vi "Compute Convex Fast Hull.vi"(2 "Bounding Rectangle (Entire Array)":T2={"Left"=-1, "Top"=-1, "Right"=-1, "Bottom"=-1}, 3 "Data":u16[][](array[numeric]), 4 "Center of Mass (0, 0)":T1) -> (0 "Interior":T1[](array[typedef]), 1 "Hull":T1[](array[typedef]))   [LabVIEW 2018, in "Video Cam Processor.lvclass"]
uses:
  Video Cam Processor.lvclass
  Private/Hull Point STYP.ctl
  Shared/Graham Scan/Graham Scan Bounding Rectangle STYP.ctl
  0152be87-d5b1-4a61-b902-843b2f58f9da.vi
  a4750f4a-c86b-4402-9379-9284bf635716.vi
  eb0064ed-dfcb-4dbb-84a7-5f2da3a78c84.vi
  2de1e9ff-1ea0-4ee2-97ee-32f0ea305ab5.vi
  ab02dc5e-4995-41ed-abd7-7908662af6ba.vi
  6afddc17-1598-4bdd-b49e-99777c4027e1.vi
  1da664a8-6403-49de-8289-c04fd4f99e1f.vi
  d6c0e748-e52f-41a4-ae1e-f13c5fdb461c.vi
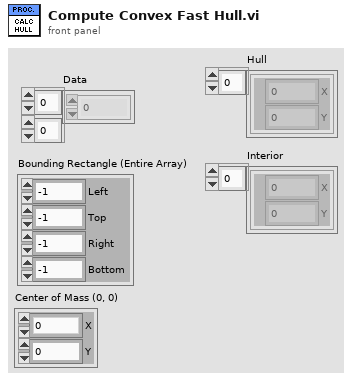
[diagram p1: front panel]
types:
  T1 = typedef "Video Cam Processor.lvclass/Hull Point STYP.ctl" = cluster{"X":i32, "Y":i32}
  T2 = typedef "Graham Scan Bounding Rectangle STYP.ctl" = cluster{"Left":i32, "Top":i32, "Right":i32, "Bottom":i32}
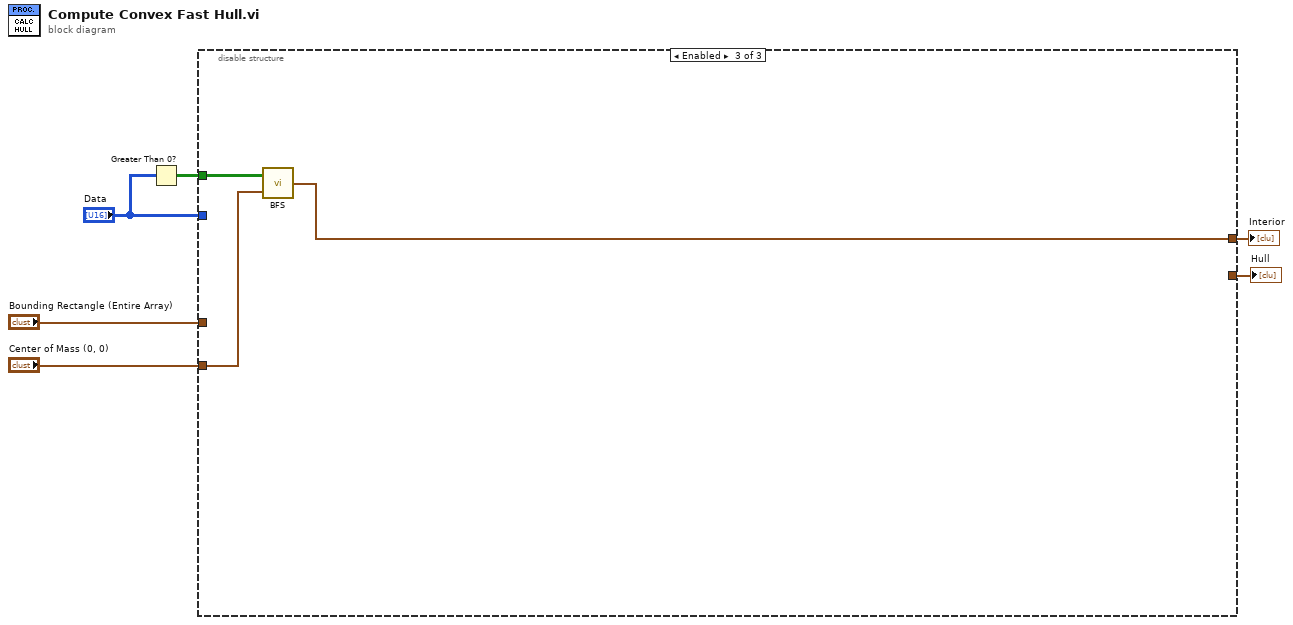
[diagram p0: block diagram]
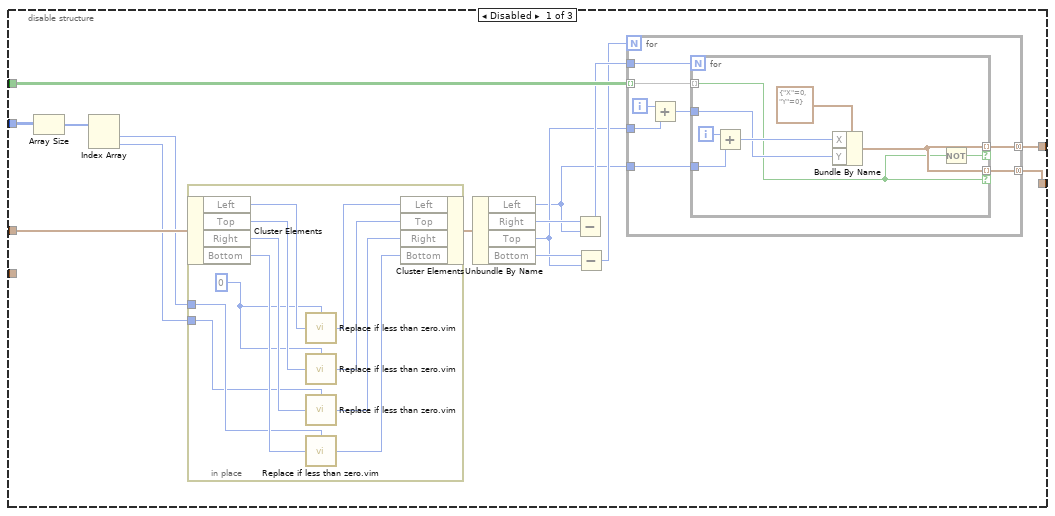
[diagram p2: hidden frame]
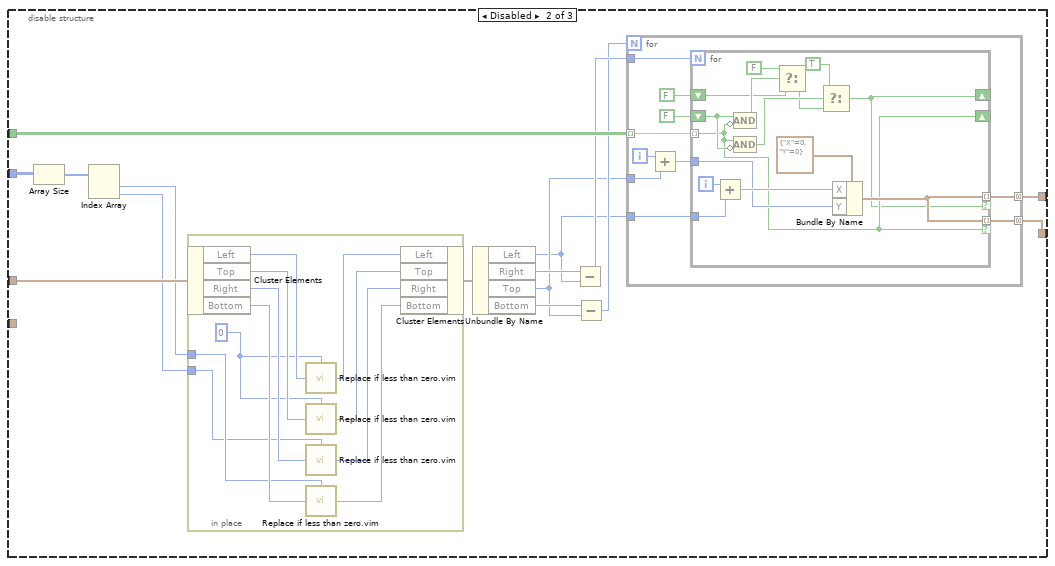
[diagram p3: hidden frame]
diagram:
  n1 = Greater Than 0?(x="Data") -> (x > 0?=w4:bool[][])
  n2 = disable-structure shown="Enabled" {
    disable-tunnel: "Bounding Rectangle (Entire Array)" -> [w20 w62 _]
    disable-tunnel: "Data" -> [w18 w60 _]
    disable-tunnel: w4 -> [w13 w55 w102]
    disable-tunnel: [w12 w54 w100] -> w3
    disable-tunnel: [w11 w53 _] -> w2
    disable-tunnel: "Center of Mass (0, 0)" -> [_ _ w101]
    frame Disabled {
      n3 = Array Size(array=w18) -> (size(s)=w21:i32[])
      n4 = Index Array(array=w21) -> (element #1=w17:i32, element #2=w16:i32)  [unwired: 2 in]
      n5 = in-place {
        in-place-border: w17 -> [w39]
        in-place-border: w16 -> [w38]
        w44 = 0
        n6 = in-place-cluster #1(w20) -> ("Left"=w48:i32, "Top"=w47:i32, "Right"=w46:i32, "Bottom"=w45:i32)
        n7 = call "Replace if less than zero.vim"("Replacement (0)"=w44, "X"=w48) -> ("Y"=w43:i32)  [unwired: 2 in]
        n8 = call "Replace if less than zero.vim"("Replacement (0)"=w44, "X"=w47) -> ("Y"=w42:i32)  [unwired: 2 in]
        n9 = call "Replace if less than zero.vim"("Replacement (0)"=w38, "X"=w46) -> ("Y"=w41:i32)  [unwired: 2 in]
        n10 = call "Replace if less than zero.vim"("Replacement (0)"=w39, "X"=w45) -> ("Y"=w40:i32)  [unwired: 2 in]
        n11 = in-place-cluster #1("Left"=w43, "Top"=w42, "Right"=w41, "Bottom"=w40) -> (w19:T2)
      }
      n12 = Unbundle By Name(w19) -> ("Left"=w7:i32, "Right"=w15:i32, "Top"=w8:i32, "Bottom"=w14:i32)
      n13 = Subtract(x=w15, y=w7) -> (x-y=w10:i32)
      n14 = Subtract(x=w14, y=w8) -> (x-y=w9:i32)
      n15 = for {
        N: w9 -> [_]
        tunnel: w13 -> [w27] mode=indexing
        tunnel: w8 -> [w28]
        tunnel: w10 -> [w26]
        tunnel: w7 -> [w25]
        tunnel: [w23] -> w12 mode=concatenating
        tunnel: [w22] -> w11 mode=concatenating
        i -> [w29]
        n16 = Add(x=w29, y=w28) -> (x+y=w24:i32)
        n17 = for {
          N: w26 -> [_]
          tunnel: w27 -> [w31] mode=indexing
          tunnel: w25 -> [w36]
          tunnel: w24 -> [w32]
          tunnel: [w34] -> w23 mode=indexing if=w30
          tunnel: [w34] -> w22 mode=indexing if=w31
          i -> [w37]
          n18 = Add(x=w37, y=w36) -> (x+y=w33:i32)
          n19 = Bundle By Name(cluster=T1 {"X"=0, "Y"=0} ("Cluster"), "X"=w33, "Y"=w32) -> (w34:T1)
          n20 = Not(x=w31) -> (.not. x?=w30:bool)
        }
      }
    }
    frame Disabled {
      n21 = Array Size(array=w60) -> (size(s)=w63:i32[])
      n22 = Index Array(array=w63) -> (element #1=w59:i32, element #2=w58:i32)  [unwired: 2 in]
      n23 = in-place {
        in-place-border: w59 -> [w90]
        in-place-border: w58 -> [w89]
        w95 = 0
        n24 = in-place-cluster #2(w62) -> ("Left"=w99:i32, "Top"=w98:i32, "Right"=w97:i32, "Bottom"=w96:i32)
        n25 = call "Replace if less than zero.vim"("Replacement (0)"=w95, "X"=w99) -> ("Y"=w94:i32)  [unwired: 2 in]
        n26 = call "Replace if less than zero.vim"("Replacement (0)"=w95, "X"=w98) -> ("Y"=w93:i32)  [unwired: 2 in]
        n27 = call "Replace if less than zero.vim"("Replacement (0)"=w89, "X"=w97) -> ("Y"=w92:i32)  [unwired: 2 in]
        n28 = call "Replace if less than zero.vim"("Replacement (0)"=w90, "X"=w96) -> ("Y"=w91:i32)  [unwired: 2 in]
        n29 = in-place-cluster #2("Left"=w94, "Top"=w93, "Right"=w92, "Bottom"=w91) -> (w61:T2)
      }
      n30 = Unbundle By Name(w61) -> ("Left"=w49:i32, "Right"=w57:i32, "Top"=w50:i32, "Bottom"=w56:i32)
      n31 = Subtract(x=w57, y=w49) -> (x-y=w52:i32)
      n32 = Subtract(x=w56, y=w50) -> (x-y=w51:i32)
      n33 = for {
        N: w51 -> [_]
        tunnel: w55 -> [w71] mode=indexing
        tunnel: w50 -> [w72]
        tunnel: w52 -> [w70]
        tunnel: w49 -> [w69]
        tunnel: [w67] -> w54 mode=concatenating
        tunnel: [w65] -> w53 mode=concatenating
        i -> [w73]
        n34 = Add(x=w73, y=w72) -> (x+y=w68:i32)
        n35 = for {
          N: w70 -> [_]
          tunnel: w71 -> [w81] mode=indexing
          tunnel: w69 -> [w87]
          tunnel: w68 -> [w83]
          tunnel: [w85] -> w67 mode=indexing if=w74
          shift-right: [w74] -> _
          shift-left: FALSE -> [w78]
          tunnel: [w85] -> w65 mode=indexing if=w81
          shift-right: [w81] -> _
          shift-left: FALSE -> [w82]
          i -> [w88]
          n36 = Add(x=w88, y=w87) -> (x+y=w84:i32)
          n37 = Compound Arithmetic op=AND(w82, invert w81) -> (w80:bool)
          n38 = Compound Arithmetic op=AND(w81, invert w82) -> (w79:bool)
          n39 = Select(t=FALSE, s=w80, f=w78) -> (s? t:f=w76:bool)
          n40 = Select(t=TRUE, s=w79, f=w76) -> (s? t:f=w74:bool)
          n41 = Bundle By Name(cluster=T1 {"X"=0, "Y"=0} ("Cluster"), "X"=w84, "Y"=w83) -> (w85:T1)
        }
      }
    }
    frame Enabled {
      n42 = call "BFS.vi"("Start (0, 0)"=w101, "Data"=w102) -> ("Valid Coordinates"=w100:T1[])
    }
  }
  "Hull" <- w2
  "Interior" <- w3
